vi "Default Color Array.vi"() -> (3 "Colors[]":u32[](array[colorbox])=[16711680, 15697664, 16776704, 6618880, 31231])   [LabVIEW 2020, in "PieChart.lvclass"]
uses:
  PieChart.lvclass
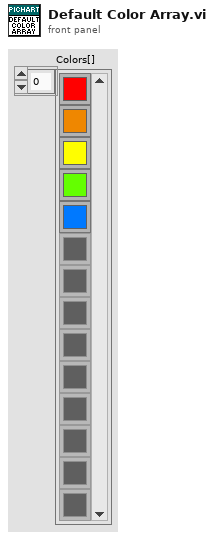
[diagram p1: front panel]
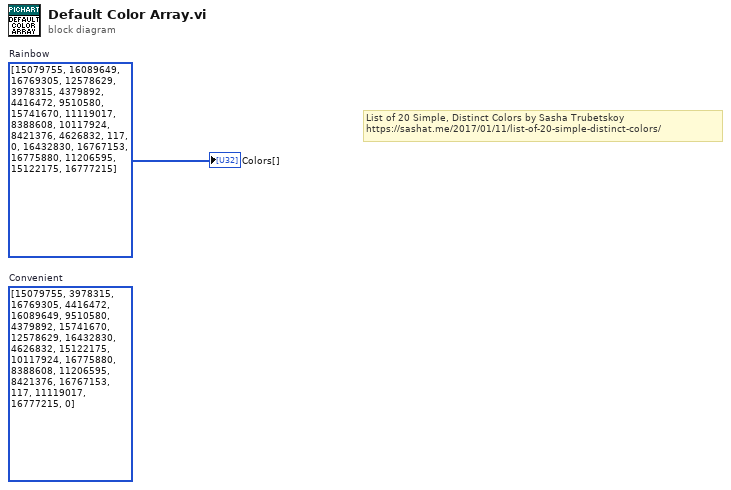
[diagram p0: block diagram]
diagram:
  (unwired) u32[] [15079755, 3978315, 16769305, 4416472, 16089649, 9510580, 4379892, 15741670, 12578629, 16432830, 4626832, 15122175, 10117924, 16775880, 8388608, 11206595, 8421376, 16767153, 117, 11119017, 16777215, 0]  # Convenient
  w1 = u32[] [15079755, 16089649, 16769305, 12578629, 3978315, 4379892, 4416472, 9510580, 15741670, 11119017, 8388608, 10117924, 8421376, 4626832, 117, 0, 16432830, 16767153, 16775880, 11206595, 15122175, 16777215]  # Rainbow
  # "List of 20 Simple, Distinct Colors by Sasha Trubetskoy\nhttps://sashat.me/2017/01/11/list-of-20-simple-distinct-colors/"
  "Colors[]" <- w1
